vi "Merge_h5_files.vi"(8 "error in (no error)":errorcluster, 10 "File to be copied in":path, 11 "Original File":path) -> (0 "error out":errorcluster)   [LabVIEW 2013]
uses:
  <vilib>/addons/h5labview/H5F_mode.ctl
  <vilib>/addons/h5labview/H5File.lvlib
  <vilib>/addons/h5labview/H5GroupObject.lvlib
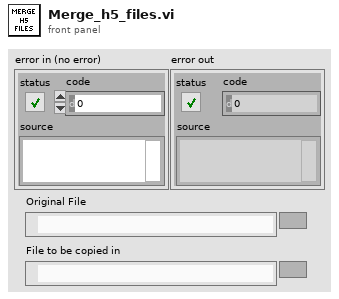
[diagram p1: front panel]
types:
  T1 = typedef "H5File.lvlib/H5F_mode.ctl" = enum16{"read-only", "read-write", "overwrite", "create new", "open or create"}
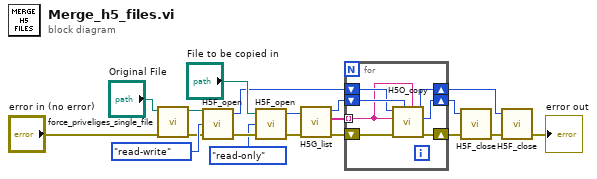
[diagram p0: block diagram]
diagram:
  n1 = call <userlib>:"force_priveliges_single_file.vi"("error in (no error)"="error in (no error)", "File path"="Original File") -> ("error out"=w4:errorcluster, "File path out"=w3:path)  [unwired: 8 in]
  n2 = call <vilib>:"H5F_open.vi"("error in (no error)"=w4, "mode"=H5F_mode."read-write", "path"=w3) -> ("error out"=w19:errorcluster, "ref"=w9:i32)  [unwired: 1 in]
  n3 = call <vilib>:"H5F_open.vi"("error in (no error)"=w19, "mode"=H5F_mode."read-only", "path"="File to be copied in") -> ("error out"=w13:errorcluster, "ref"=w14:i32)  [unwired: 1 in]
  n4 = call <vilib>:"H5G_list.vi"("error in (no error)"=w13, "ref"=w14) -> ("error out"=w11:errorcluster, "names"=w12:string[], "ref out"=w10:i32)  [unwired: 2 in, 1 out]
  n5 = for {
    tunnel: w12 -> [w22] mode=indexing
    shift-right: [w25] -> w8
    shift-left: w11 -> [w26]
    shift-right: [w21] -> w7
    shift-left: w10 -> [w24]
    shift-right: [w20] -> w6
    shift-left: w9 -> [w23]
    n6 = call <vilib>:"H5O_copy.vi"("src_name"=w22, "src_id"=w24, "error in (no error)"=w26, "dest_name"=w22, "dest_id"=w23) -> ("error out"=w25:errorcluster, "src out"=w21:i32, "dest out"=w20:i32)  [unwired: 4 in]
  }
  n7 = call <vilib>:"H5F_close.vi"("error in (no error)"=w8, "ref"=w7) -> ("error out"=w15:errorcluster)  [unwired: 3 in]
  n8 = call <vilib>:"H5F_close.vi"("error in (no error)"=w15, "ref"=w6) -> ("error out"=→"error out":errorcluster)  [unwired: 3 in]
